vi "4461 - AI AND AI - Read AND Write Uneven - SINGLE TASK.vi"(6 "AO Array":waveform(dbl)[](array[waveform]), 8 "error in (no error)":errorcluster, 10 "AO task":refnum<k21>, 11 "AI task":refnum<k21>) -> (0 "error out":errorcluster, 3 "AI Read":waveform(dbl)[](array[waveform]))   [LabVIEW 2016]
uses:
  <vilib>/DAQmx/write.llb/DAQmx Write (Analog 1D Wfm NChan NSamp).vi
  <vilib>/DAQmx/read.llb/DAQmx Read (Analog 1D Wfm NChan NSamp).vi
  <vilib>/DAQmx/miscellaneous.llb/DAQmx Fill In Error Info.vi
  <resource>/objmgr/daqmx.rc
panel:
  in  "Sampling Stuff (AI & AO)":T1={"sampling info"={"Fs"=0.0, "#s"=0.0}, "sample mode"=10178, "AI Buffer Size (S)"=10} {"sample mode" items=["Finite Samples"=10178, "Continuous Samples"=10123]}
  out "Numeric":i32
  out "AvailSampPerChan":u32
  # "AI (READ) AND AO (WRITE)"
  # "OUTPUTS"
  # "INPUTS"
  # "These are just for debugging / monitoring"
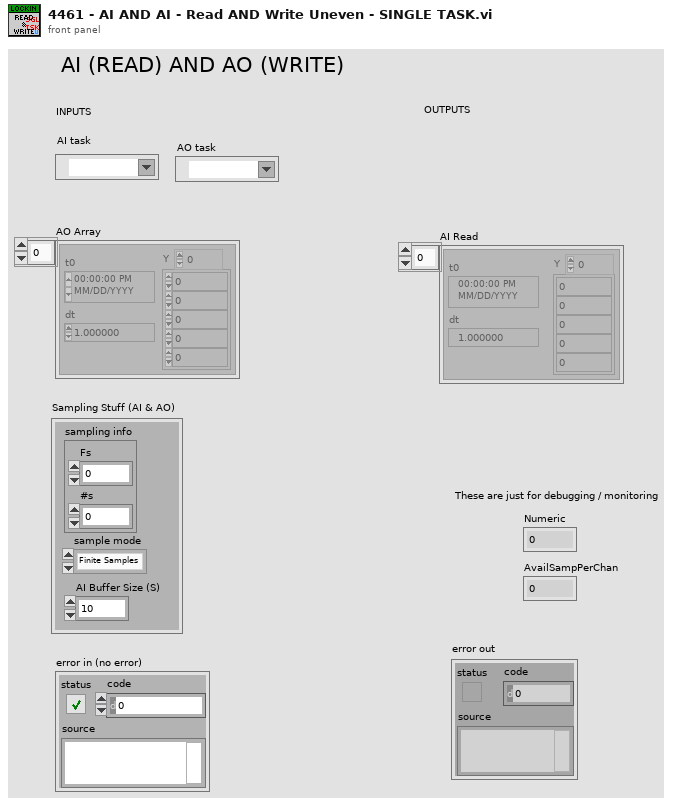
[diagram p1: front panel]
types:
  T1 = cluster{"sampling info":cluster{"Fs":dbl, "#s":dbl}, "sample mode":i32, "AI Buffer Size (S)":i32}
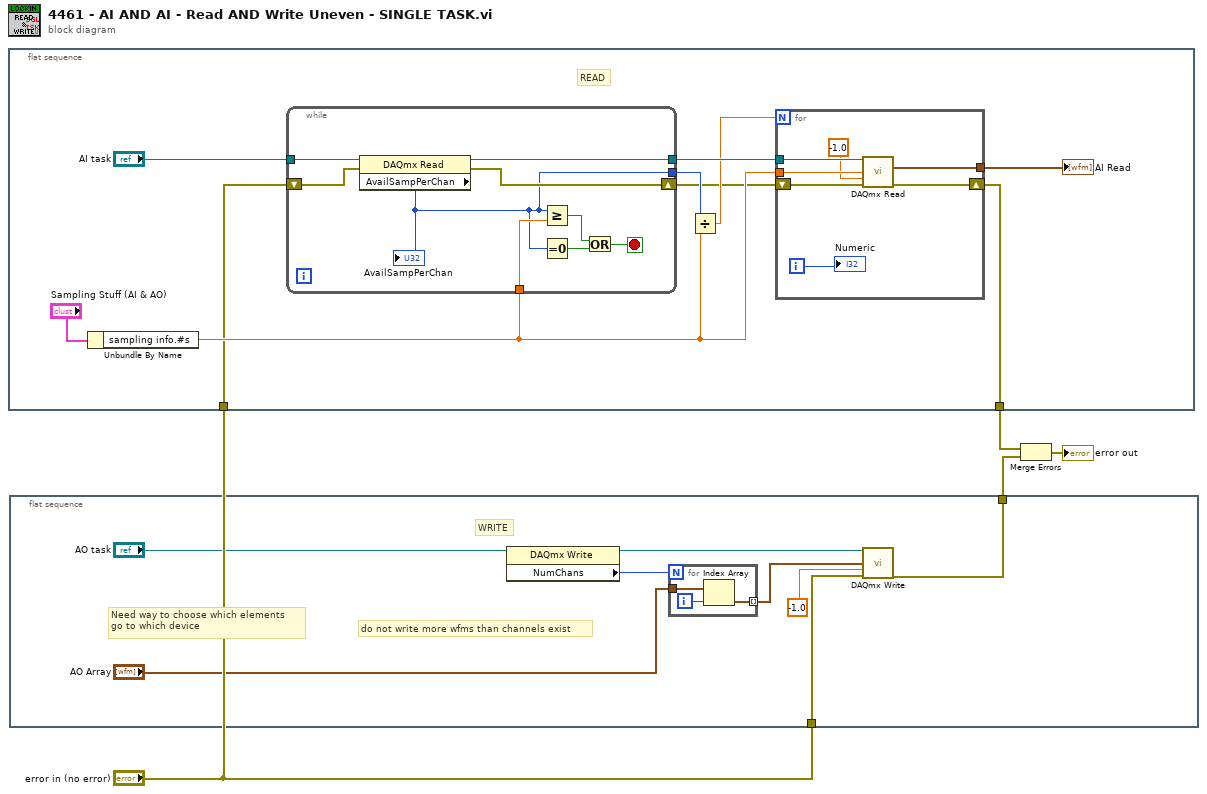
[diagram p0: block diagram]
diagram:
  n1 = flat-sequence {
    tunnel: "error in (no error)" -> [w7]
    tunnel: [w6] -> w3
    frame #0 {
      # "READ"
      n2 = Unbundle By Name("Sampling Stuff (AI & AO)") -> ("sampling info.#s"=w14:dbl)
      n3 = while {
        tunnel: [w30] -> w13
        tunnel: w14 -> [w28]
        tunnel: [w23] -> w11
        tunnel: "AI task" -> [w24]
        shift-right: [w29] -> w8
        shift-left: w7 -> [w22]
        stop <- w27 stop-if-true
        n4 = property class="DAQmx Read"(reference=w24, error in=w22) -> (reference out=w30:refnum<k21>, error out=w29:errorcluster, "AvailSampPerChan"=w23:u32)
        "AvailSampPerChan" <- w23
        n5 = Greater Or Equal?(x=w23, y=w28) -> (x >= y?=w25:bool)
        n6 = Equal To 0?(x=w23) -> (x = 0?=w26:bool)
        n7 = Or(x=w25, y=w26) -> (x .or. y?=w27:bool)
      }
      n8 = Divide(x=w11, y=w14) -> (x/y=w12:dbl)
      n9 = for {
        N: w12 -> [_]
        tunnel: w13 -> [w21]
        tunnel: [w20] -> w9
        tunnel: w14 -> [w19]
        shift-right: [w18] -> w6
        shift-left: w8 -> [w15]
        i -> [w17]
        n10 = call-poly <vilib>:"DAQmx Read.vi"("task/channels in"=w21, "number of samples per channel"=w19, "timeout"=-1.0, "error in"=w15) -> ("data"=w20:waveform(dbl)[], "error out"=w18:errorcluster)  [unwired: 9 in, 1 out]
        "Numeric" <- w17
      }
      "AI Read" <- w9
    }
  }
  n11 = flat-sequence {
    tunnel: [w34] -> w2
    tunnel: "error in (no error)" -> [w31]
    frame #0 {
      # "Need way to choose which elements\ngo to which device"
      # "WRITE"
      # "do not write more wfms than channels exist"
      n12 = property class="DAQmx Write"(reference="AO task") -> (reference out=w36:refnum<k21>, "NumChans"=w38:u32)  [unwired: 1 in, 1 out]
      n13 = for {
        N: w38 -> [_]
        tunnel: "AO Array" -> [w41]
        tunnel: [w40] -> w33 mode=indexing
        i -> [w39]
        n14 = Index Array(array=w41, index=w39) -> (element=w40:waveform(dbl))
      }
      n15 = call-poly <vilib>:"DAQmx Write.vi"("task/channels in"=w36, "data"=w33, "timeout"=-1.0, "error in"=w31) -> ("error out"=w34:errorcluster)  [unwired: 9 in, 2 out]
    }
  }
  n16 = Merge Errors(w3, w2) -> (→"error out":errorcluster)
